vi "SendPN2PLC.vi"(8 "error in (no error)":errorcluster, 10 "Station":string, 11 "PN":string) -> (0 "error out":errorcluster, 2 "Result":string)   [LabVIEW 2020]
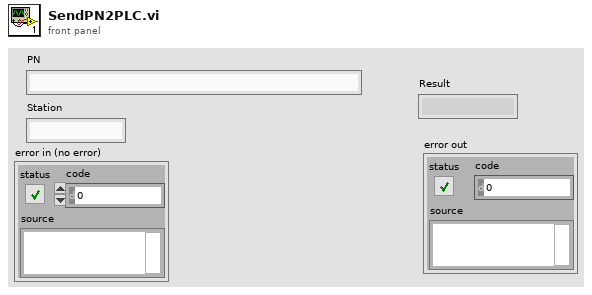
[diagram p1: front panel]
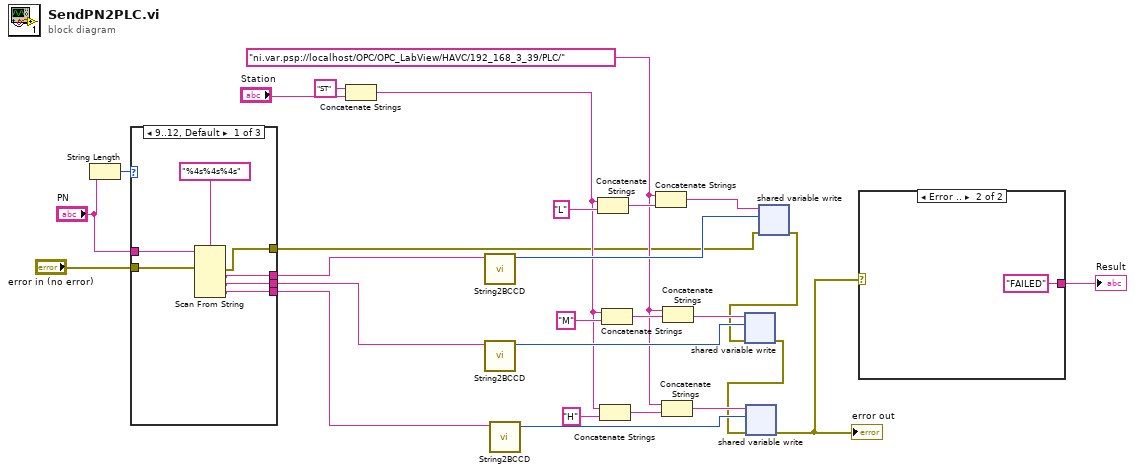
[diagram p0: block diagram]
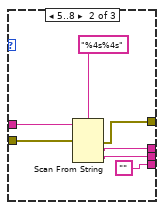
[diagram p2: hidden frame]
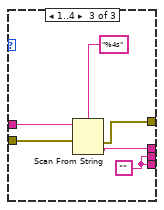
[diagram p3: hidden frame]
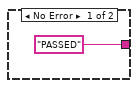
[diagram p4: hidden frame]
diagram:
  w17 = "ni.var.psp://localhost/OPC/OPC_LabView/HAVC/192_168_3_39/PLC/" ("string")
  n1 = String Length(string="PN") -> (length=w7:i32)
  n2 = case shown="9..12, Default" w7 {
    tunnel: "PN" -> [w33 w40 w46]
    tunnel: "error in (no error)" -> [w32 w39 w45]
    tunnel: [w31 w38 w44] -> w4
    tunnel: [w30 w37 w43] -> w3
    tunnel: [w29 w36 w42] -> w2
    tunnel: [w28 "" w42] -> w1
    frame 9..12, Default {
      n3 = Scan From String(format string="%4s%4s%4s", input string=w33, error in=w32) -> (error out=w31:errorcluster, output 1=w30:string, output 2=w29:string, output 3=w28:string)  [unwired: 4 in, 2 out]
    }
    frame 5..8 {
      n4 = Scan From String(format string="%4s%4s", input string=w40, error in=w39) -> (error out=w38:errorcluster, output 1=w37:string, output 2=w36:string)  [unwired: 3 in, 2 out]
    }
    frame 1..4 {
      w42 = ""
      n5 = Scan From String(format string="%4s", input string=w46, error in=w45) -> (error out=w44:errorcluster, output 1=w43:string)  [unwired: 2 in, 2 out]
    }
  }
  n6 = Concatenate Strings("ST" ("string"), "Station") -> (w15:string)
  n7 = call "String2BCCD.vi"("String"=w3) -> ("BCD Int"=w26:i64)  [unwired: 10 in]
  n8 = call "String2BCCD.vi"("String"=w2) -> ("BCD Int"=w24:i64)  [unwired: 10 in]
  n9 = call "String2BCCD.vi"("String"=w1) -> ("BCD Int"=w13:i64)  [unwired: 10 in]
  n10 = Concatenate Strings(w15, "L" ("string")) -> (w22:string)
  n11 = Concatenate Strings(w15, "H" ("string")) -> (w18:string)
  n12 = Concatenate Strings(w15, "M" ("string")) -> (w21:string)
  n13 = Concatenate Strings(w17, w22) -> (w27:string)
  n14 = Concatenate Strings(w17, w18) -> (w16:string)
  n15 = Concatenate Strings(w17, w21) -> (w25:string)
  n16 = shared-variable-write(w27, w4, w26) -> (w11:errorcluster)  [unwired: 1 out]
  n17 = shared-variable-write(w25, w11, w24) -> (w10:errorcluster)  [unwired: 1 out]
  n18 = shared-variable-write(w16, w10, w13) -> (w9:errorcluster)  [unwired: 1 out]
  "error out" <- w9
  n19 = case shown="Error .." w9 {
    tunnel: ["PASSED" "FAILED"] -> w8
    frame No Error {
    }
    frame Error {
    }
  }
  "Result" <- w8
